vi "LVClass_ModalCoef Get Dimension Coef map.vi"(0 "ModalCoef in":refnum<class "ModalCoef.lvclass">, 11 "error in (no error)":errorcluster) -> (4 "ModalCoef out":refnum<class "ModalCoef.lvclass">, 6 "# of coef":i32, 15 "error out":errorcluster)   [LabVIEW 2020, in "ModalCoef.lvclass"]
doc: "Retrieve polynomial coefficients count.\n\n--------------------------------------------------------------------------------\n\n<B>TypePhaseIn </B> : TypePhase phase mode reconstruction.\n<B>TypePhaseOut </B> : TypePhase phase mode reconstruction.\n<B>modalCoef </B> : ModalCoef object.\n<B>size </B> : Number of modal coefficients.\n<B>ErrorIn </B> : Error\n<B>ErrorOut </B> : Error\n\n--------------------------------------------------------------------------------"
uses:
  ModalCoef.lvclass
  ModalCoef.lvclass/ModalCoef.ctl
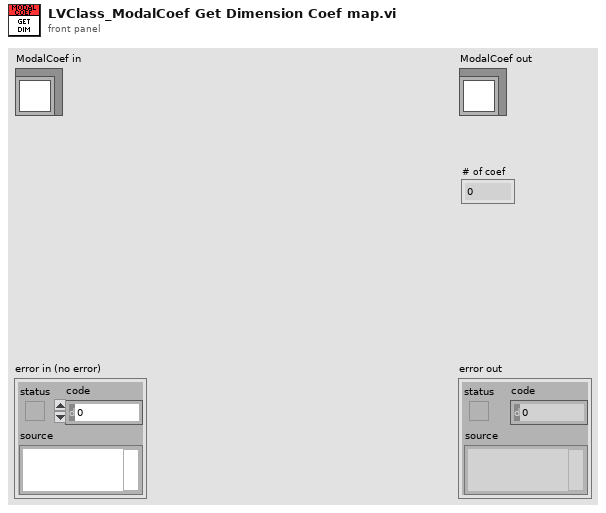
[diagram p1: front panel]
types:
  T1 = typedef "ClassID.ctl" = i64
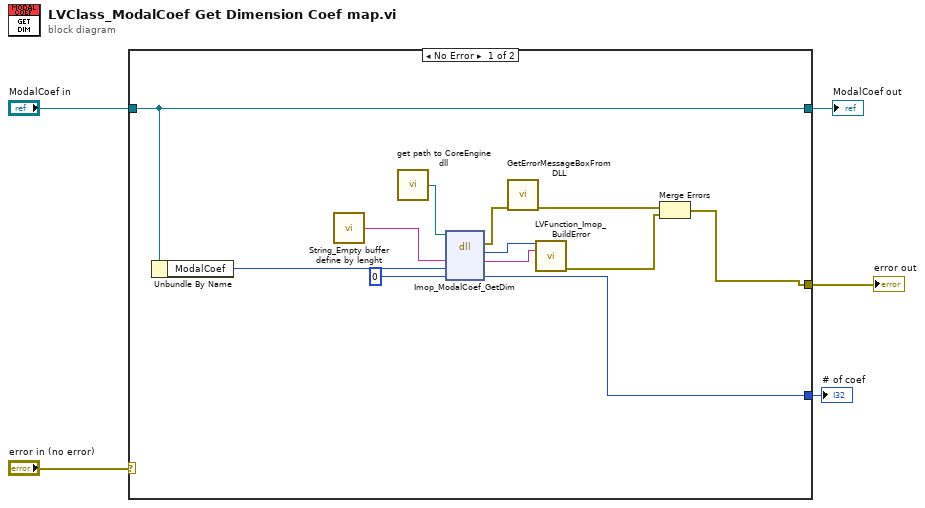
[diagram p0: block diagram]
diagram:
  n1 = case shown="No Error" "error in (no error)" {
    selector: "error in (no error)" -> [_ w19]
    tunnel: [w7 w19] -> w4
    tunnel: [w16 w18] -> w2
    tunnel: "ModalCoef in" -> [w16 w18]
    tunnel: [w10 _] -> w1
    frame No Error {
      n2 = Unbundle By Name(w16) -> ("ModalCoef"=w17:T1)
      n3 = call "String_Empty buffer define by lenght.vi"() -> ("Empty buffer"=w15:string)  [unwired: 1 in]
      n4 = call "get path to CoreEngine dll.vi"() -> ("path to wavekit library"=w12:path)  [unwired: 14 in, 1 out]
      n5 = dll-call lib="D:/2_trunk/Soft_haso/ImOpCoreEngine4_LV2011/DLLs/ImopEngine4_vc100.dll" fn="Imop_ModalCoef_GetDim"(path in=w12, "message"=w15, "ModalCoefs"=w17, "size"=u32 0 ("coef")) -> (error out=w11:errorcluster, "return type"=w13:i32, "message"=w14:string, "size"=w10:u32)  [unwired: 3 in, 1 out]
      n6 = call "GetErrorMessageBoxFromDLL.vi"("error IN"=w11) -> ("error OUT"=w9:errorcluster)  [unwired: 10 in]
      n7 = call "LVFunction_Imop_BuildError.vi"("code"=w13, "String to Prepend to source (\"\")"=w14) -> ("error out"=w8:errorcluster)  [unwired: 13 in]
      n8 = Merge Errors(w9, w8) -> (w7:errorcluster)
    }
    frame Error {
    }
  }
  "error out" <- w4
  "ModalCoef out" <- w2
  "# of coef" <- w1
